vi "Main.vi"(0 "Search Bar":string(combo), 1 "Copy":bool, 2 "Expand/Collapse All":bool, 5 "Tree":string[](tree), 7 "Top Level folder path":path, 11 "Error In":errorcluster) -> (4 "Path":path, 6 "Report String":string, 15 "Error Out":errorcluster)   [LabVIEW 2019]
doc: "Implements a file explorer interface to display folders and files, displaying attributes and supporting operations like selection, copying, sorting and report generation about the folders."
uses:
  Controls/Queue Operation.ctl
  Controls/Queue Element.ctl
  Controls/File explorer Data.ctl
  Controls/Item.ctl
  <vilib>/Utility/miscctls.llb/LVPoint32TypeDef.ctl
  49cb5066-c8fb-45b1-b1e9-3b55b32f25bf.vi
  Controls/Error Details.ctl
panel:
  # "Instructions:\n1. Run the VI.\n2. Specify the top-level folder path and view the folder structure along with its attributes in the tree control.\n3. Tree headers acts as sorting triggers.\n4. Click the checkbox next to folder to select or deselect it. View the generated report for the checked folders in the report string.\n5. Press the Expand/Collapse button to expand/collapse all the items in the tree.\n6. Enter the folder name in the search bar to expand all the nodes that match the searched keyword.\n7. Select the files and click on the copy to copy the files in the desired destination.\n8. Click Panel Close to stop the VI."
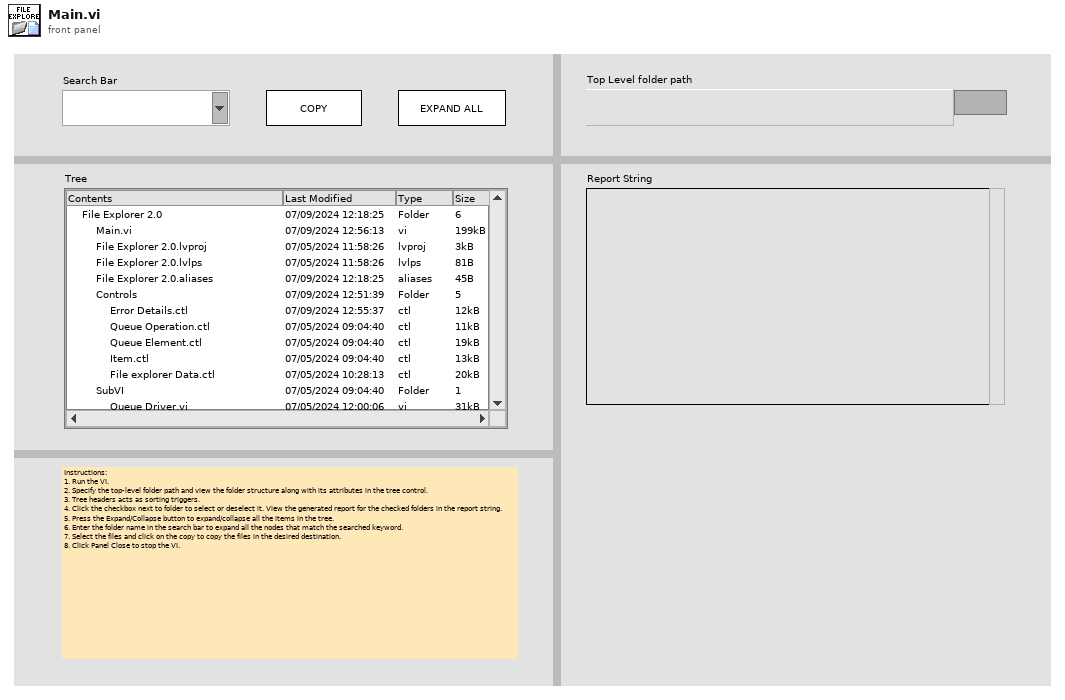
[diagram p1: front panel]
types:
  T1 = typedef "Queue Element.ctl" = cluster{"State":string, "Data":variant}
  T2 = typedef "File explorer Data.ctl" = cluster{"Path In":path, "Indent":i32, "All Folders":path[], "All Files":path[], "Folder Items":T3[], "File Items":T3[], "Selected tags":string[], "Report String":string, "Search String":string, "Search Results":string[], "Checked Folders":string[], "Files Selected":string[], "Stop Event":refnum<user-event>, "Sort Header":i32, "Time Flag":i16, "Type Flag":i16, "Size Flag":i16, "Reverse?":bool, "New Folder Path":path, "Expand?":bool, "Open? State":bool[], "Nodes":path[], "Active Tag":string, "Repopulate?":bool}
  T3 = typedef "Item.ctl" = cluster{"Left Cell String":string, "Child Text":string[], "Child Tag":string, "Child Only?":bool, "Parent Tag":string, "Item Indent":i32}
  T4 = typedef "Queue Operation.ctl" = enum16{"Create and Enqueue N", "Enqueue", "Enqueue N", "Dequeue", "Enstack N", "Flush", "Release"}
  T5 = typedef "LVPoint32TypeDef.ctl" = cluster{"Horizontal":i32, "Vertical":i32}
  T6 = typedef "Error Details.ctl" = errorcluster
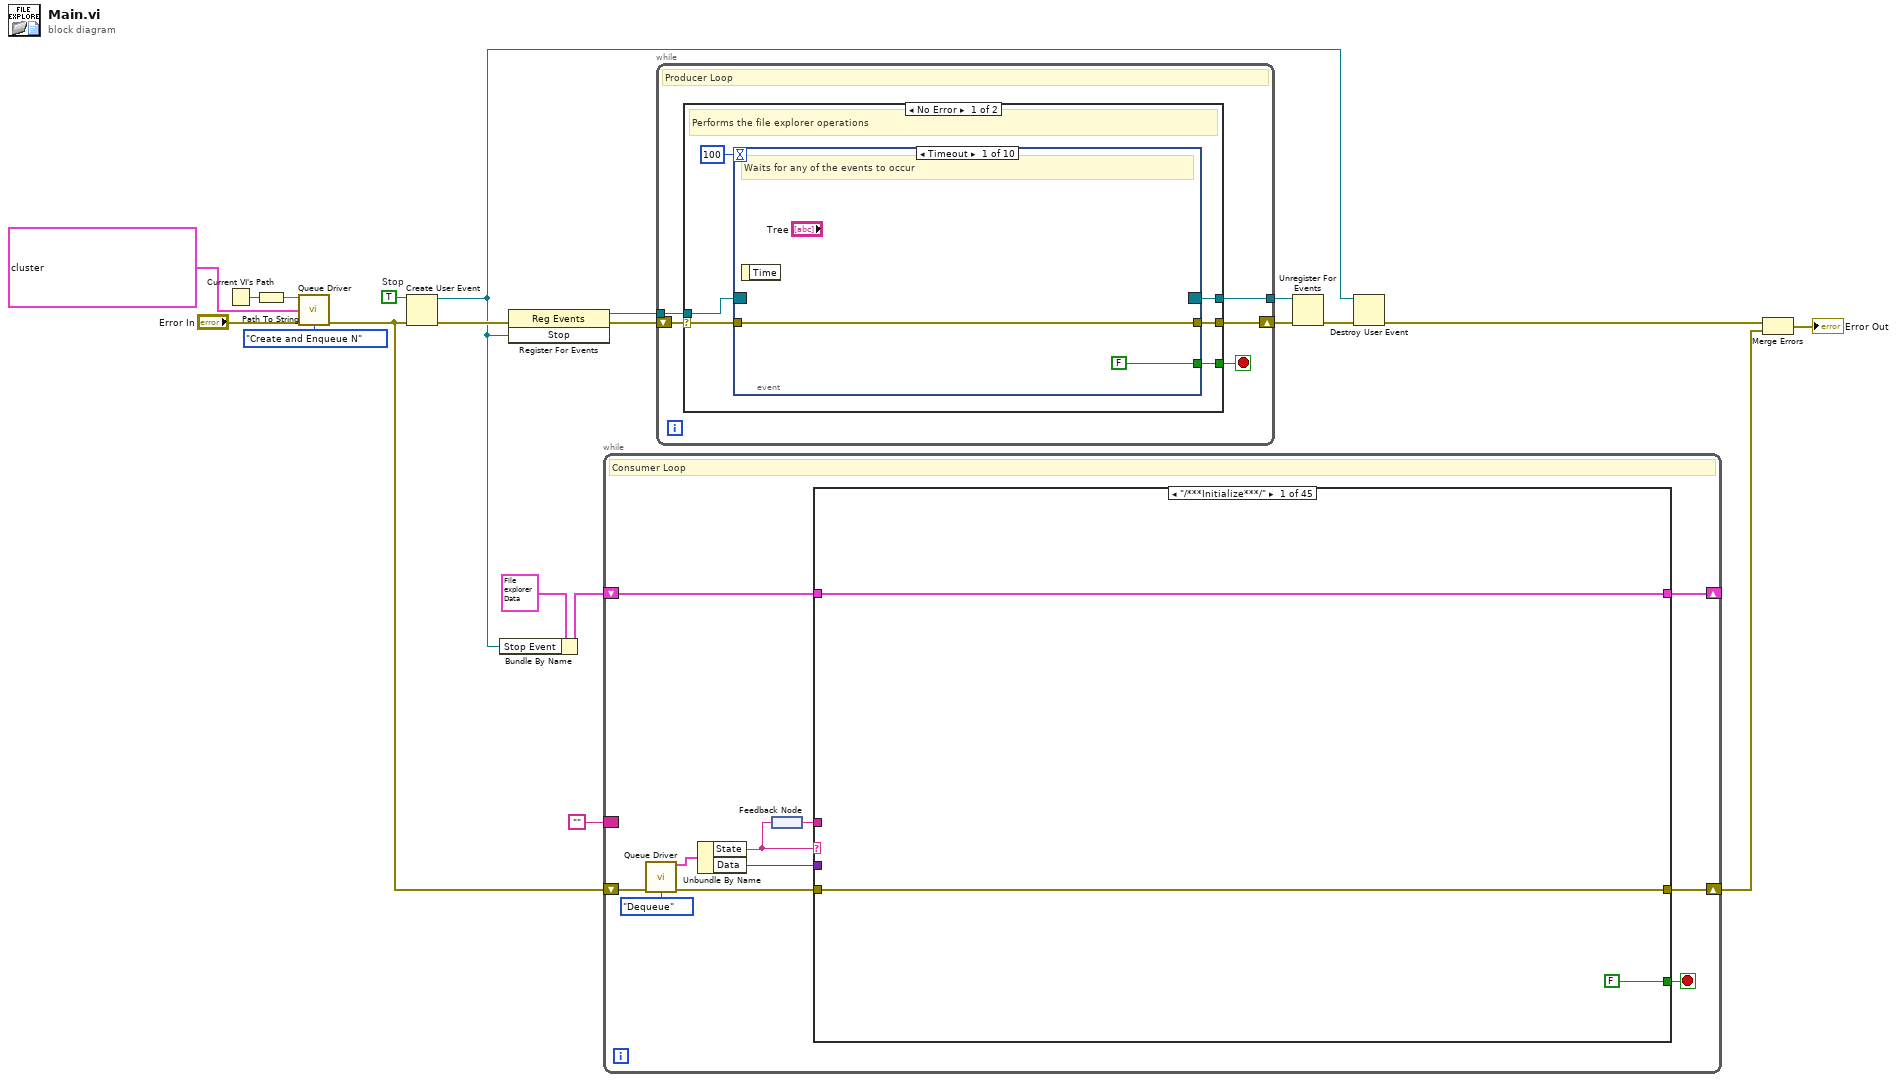
[diagram p0: block diagram]
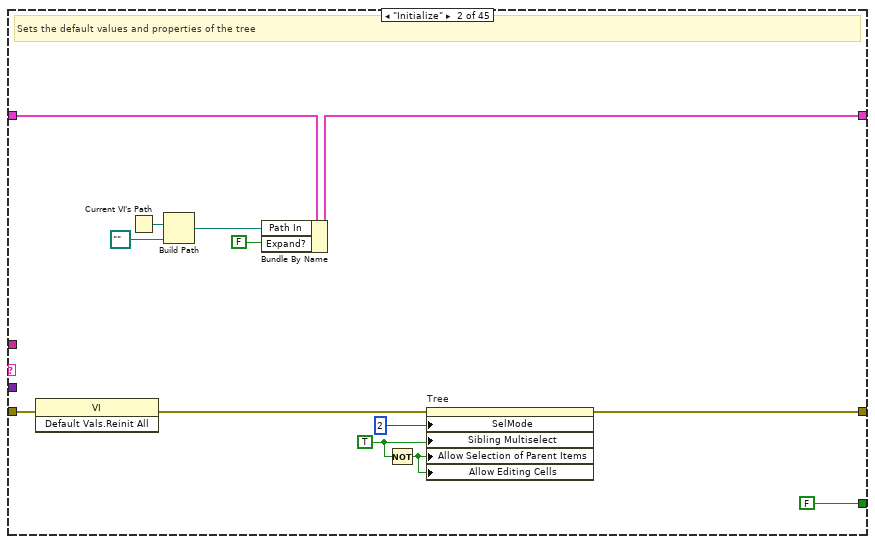
[diagram p2: hidden frame]
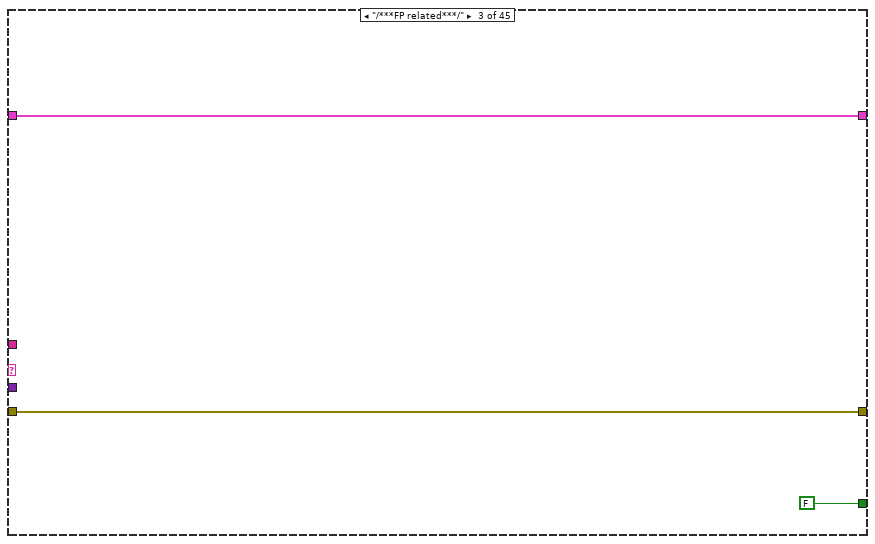
[diagram p3: hidden frame]
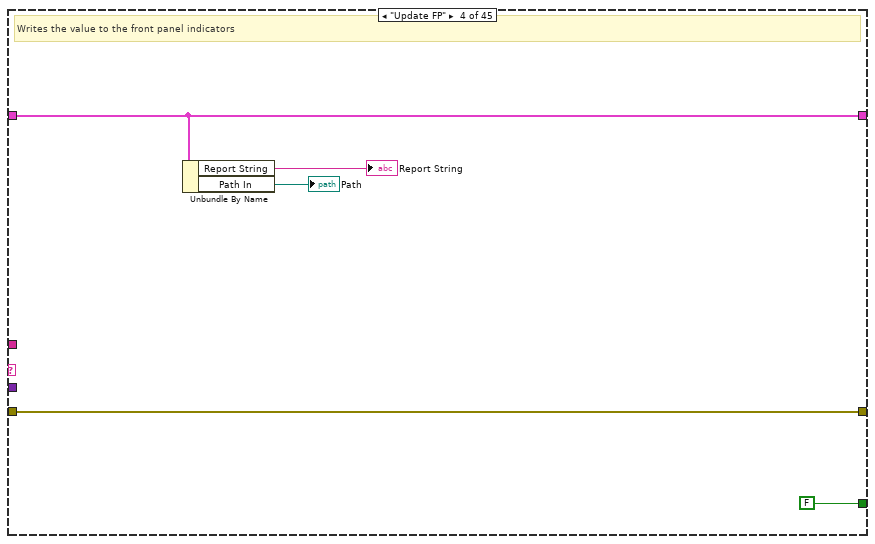
[diagram p4: hidden frame]
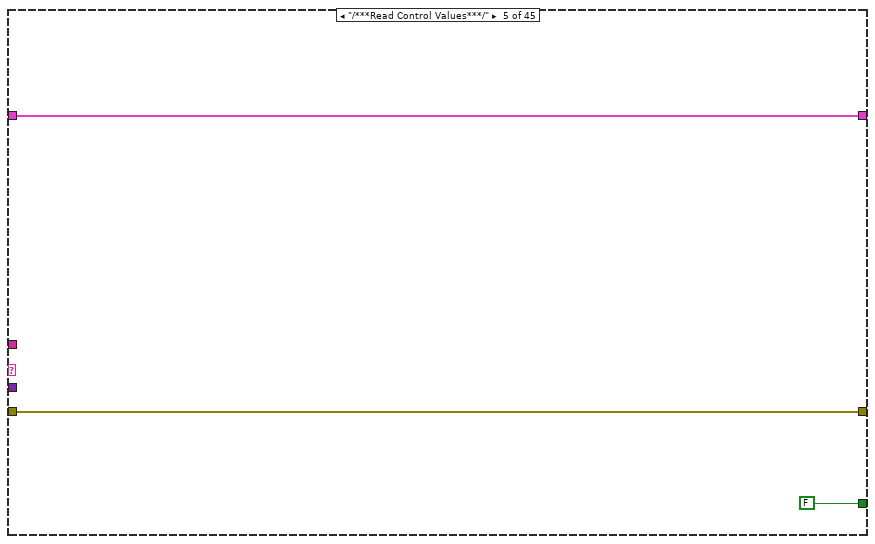
[diagram p5: hidden frame]
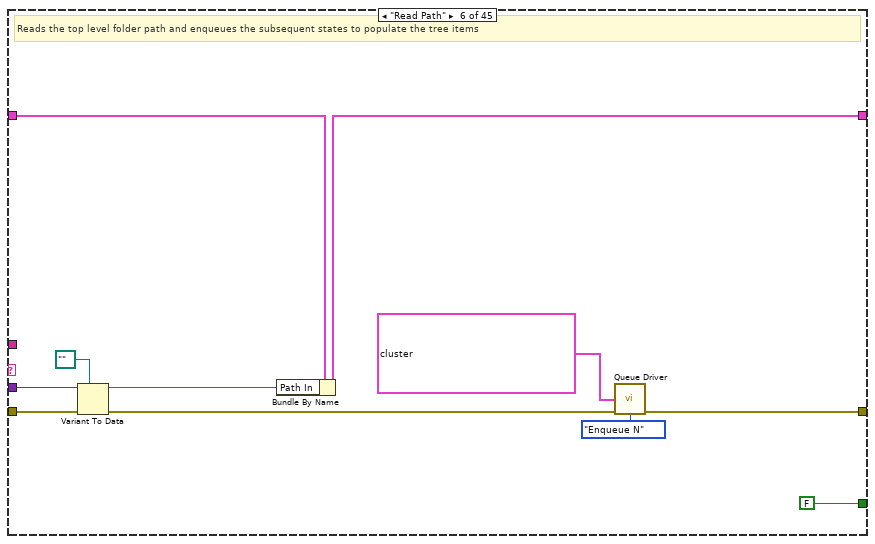
[diagram p6: hidden frame]
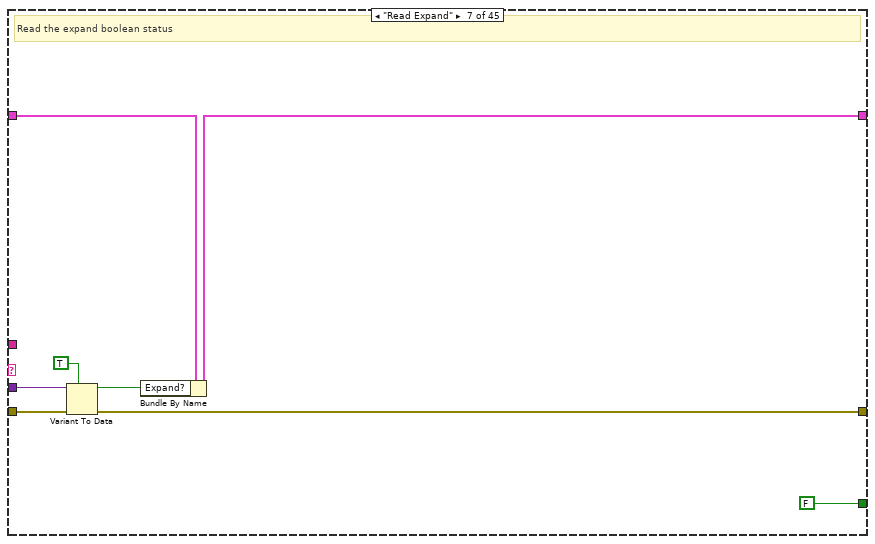
[diagram p7: hidden frame]
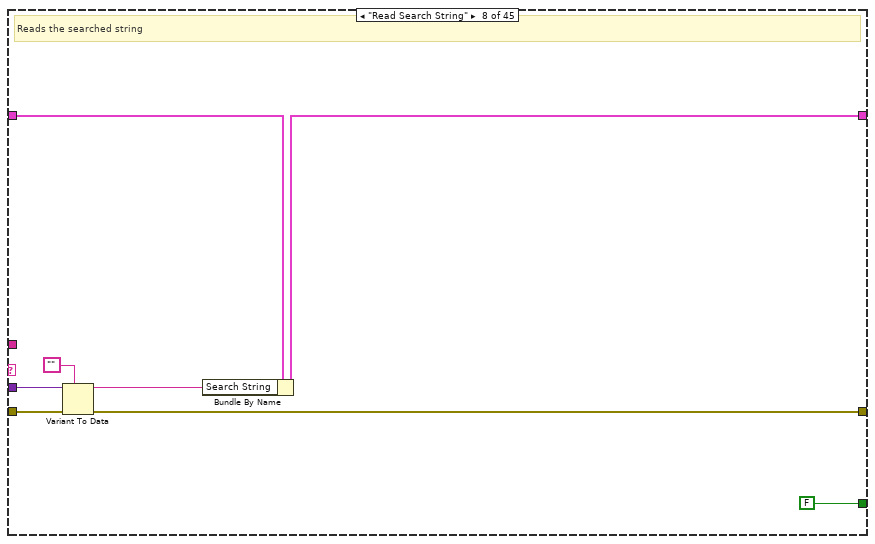
[diagram p8: hidden frame]
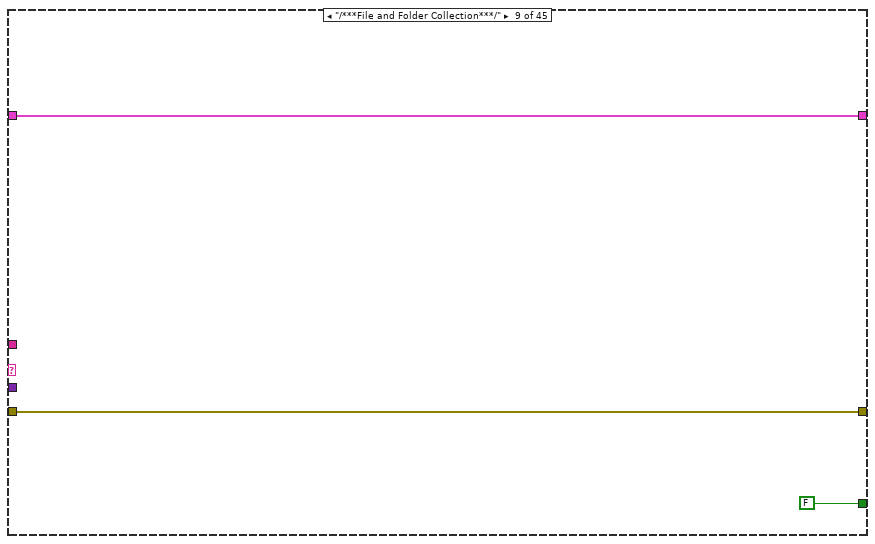
[diagram p9: hidden frame]
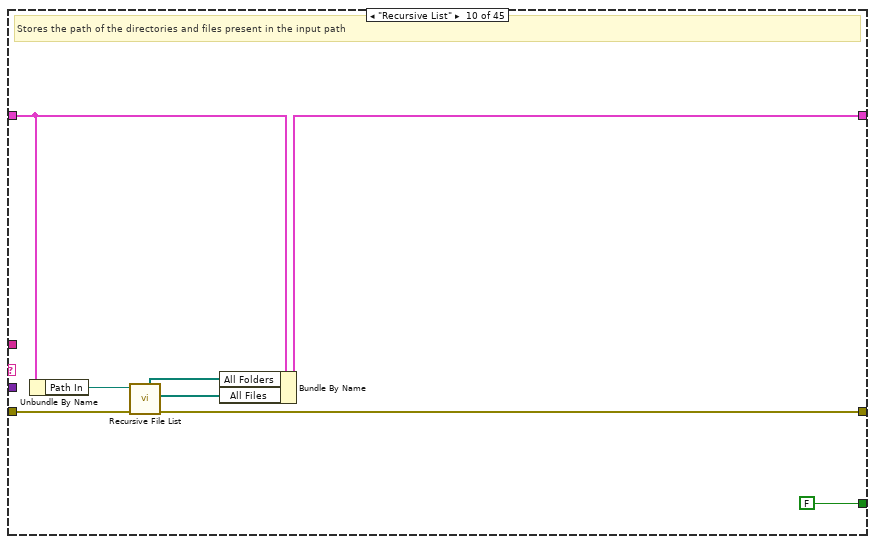
[diagram p10: hidden frame]
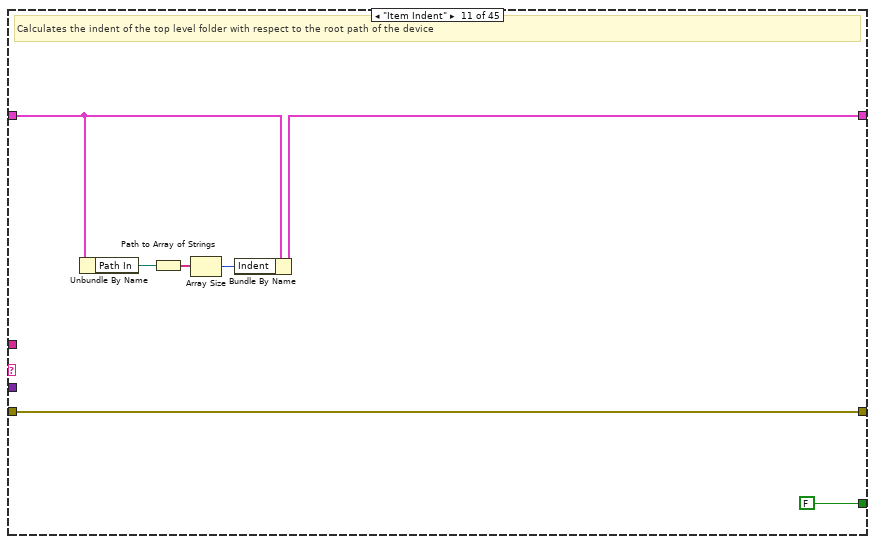
[diagram p11: hidden frame]
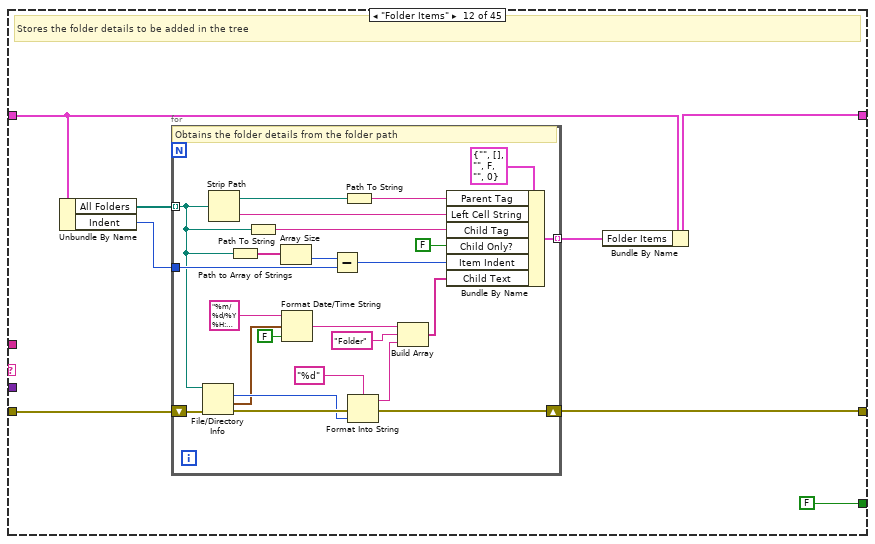
[diagram p12: hidden frame]
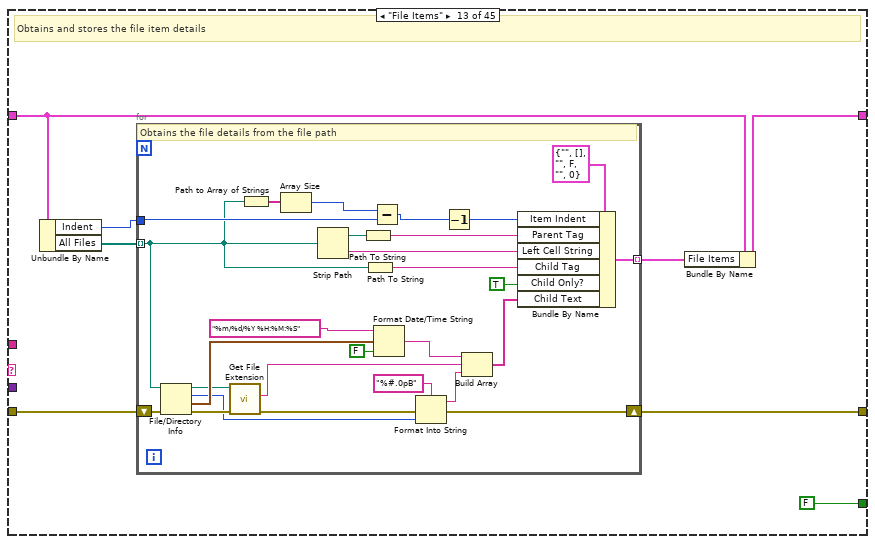
[diagram p13: hidden frame]
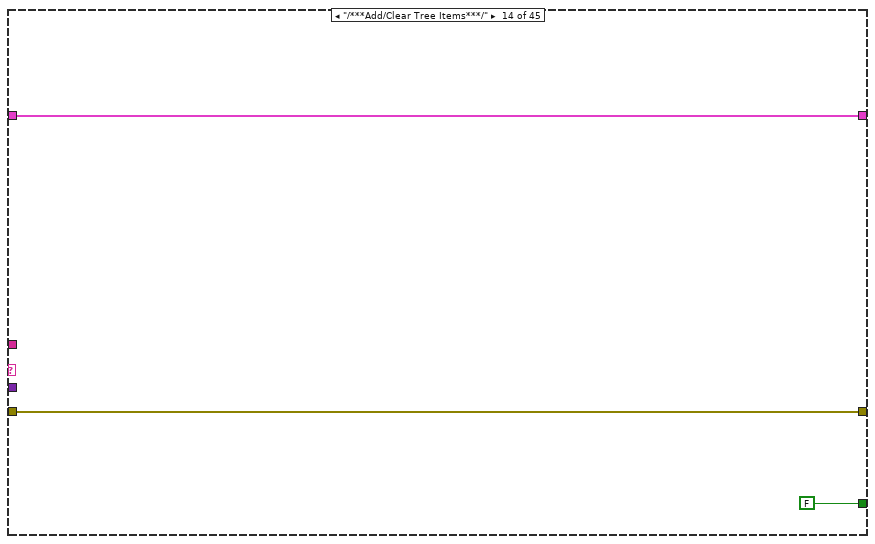
[diagram p14: hidden frame]
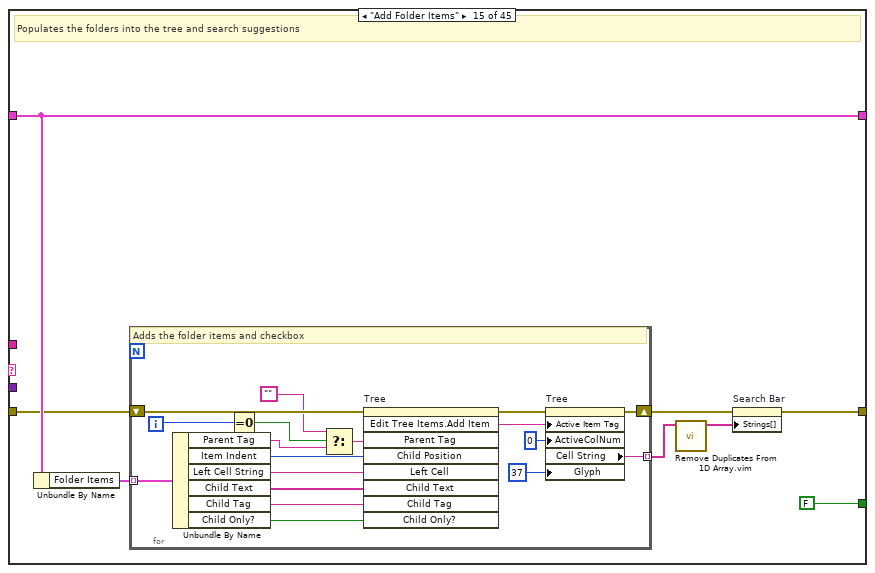
[diagram p15: hidden frame]
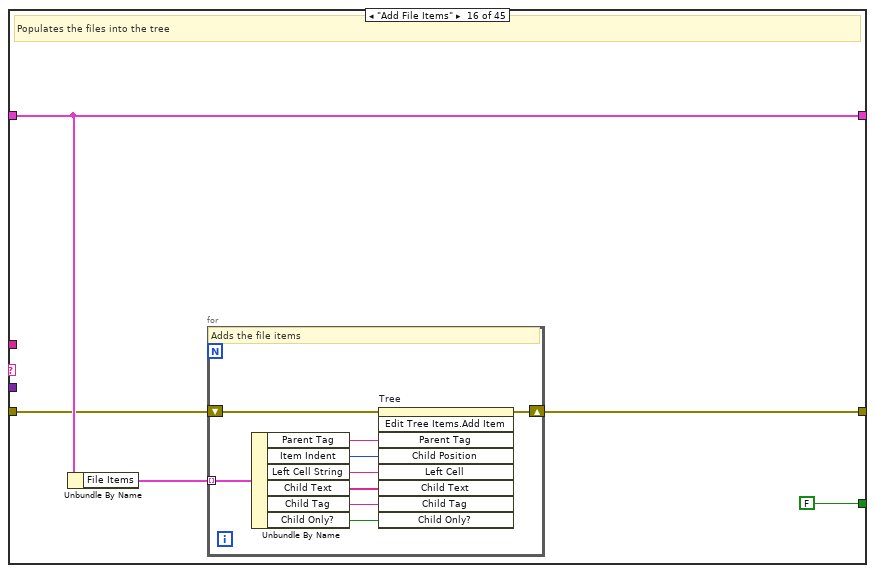
[diagram p16: hidden frame]
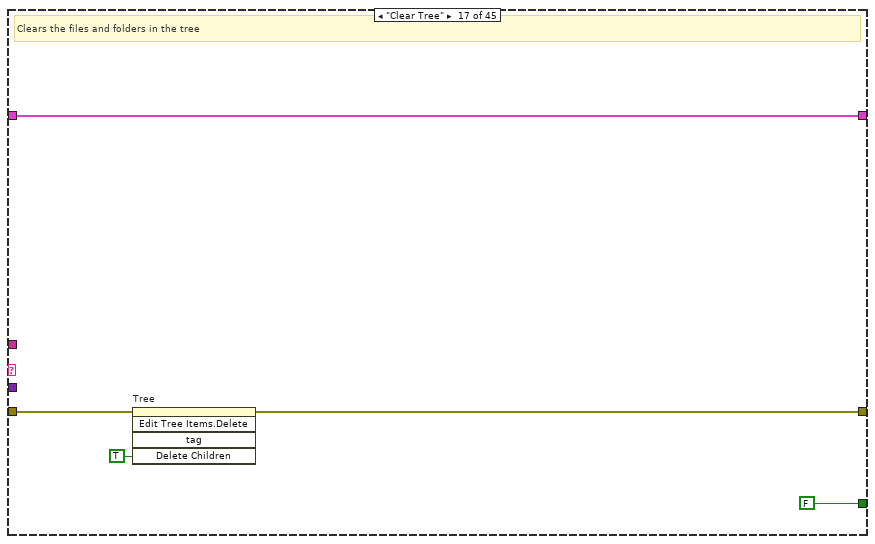
[diagram p17: hidden frame]
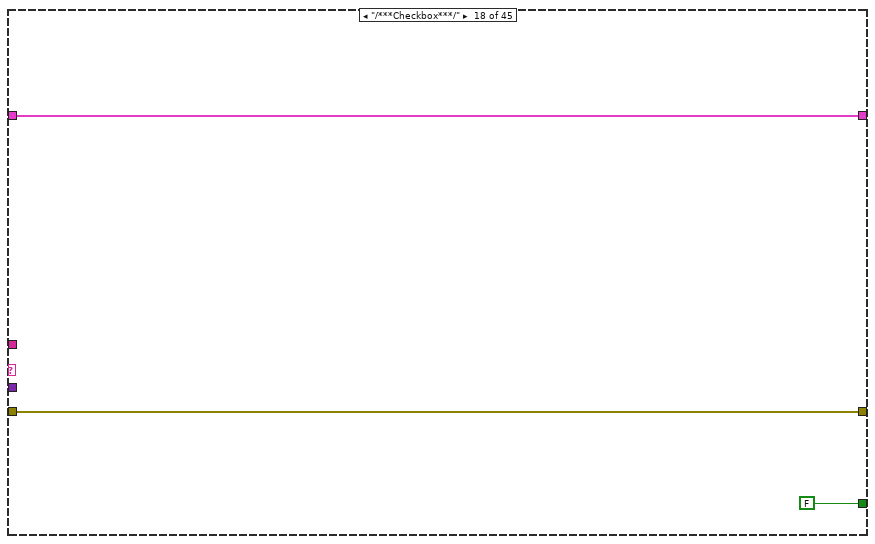
[diagram p18: hidden frame]
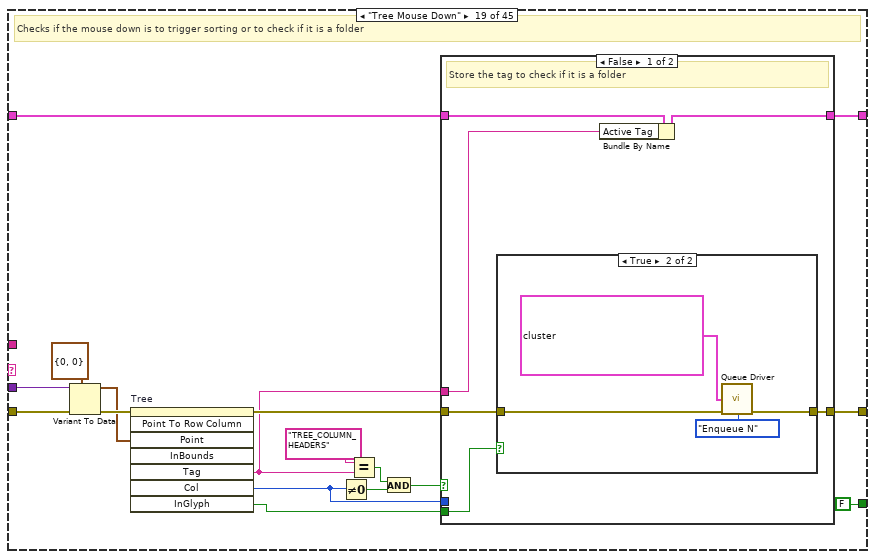
[diagram p19: hidden frame]
diagram:
  w11 = TRUE  # Stop
  n1 = Current VI's Path() -> (path=w3:path)
  n2 = Path To String(path=w3) -> (string=w2:string)
  n3 = call "Queue Driver.vi"("Queue Name"=w2, "Array of Elements"=T1[] [{"State"="Initialize", "Data"=variant}, {"State"="Update FP", "Data"=variant}, {"State"="Clear Tree", "Data"=variant}, {"State"="Recursive List", "Data"=variant}, {"State"="Item Indent", "Data"=variant}, {"State"="Folder Items", "Data"=variant}, {"State"="File Items", "Data"=variant}, {"State"="Add Folder Items", "Data"=variant}, {"State"="Expand or Collapse", "Data"=variant}, {"State"="Add File Items", "Data"=variant}], "Error In"="Error In", "Queue Operation"=Queue_Operation."Create and Enqueue N") -> ("Error Out"=w17:errorcluster)  [unwired: 10 in, 1 out]
  n4 = Create User Event(user event datatype=w11, error in=w17) -> (user event=w4:refnum<user-event>, error out=w12:errorcluster)
  n5 = Bundle By Name(cluster=T2 {"Path In"=path "", "Indent"=0, "All Folders"=[], "All Files"=[], "Folder Items"=[], "File Items"=[], "Selected tags"=[], "Report String"="", "Search String"="", "Search Results"=[], "Checked Folders"=[], "Files Selected"=[], "Stop Event"=refnum, "Sort Header"=0, "Time Flag"=0, "Type Flag"=0, "Size Flag"=0, "Reverse?"=TRUE, "New Folder Path"=path "", "Expand?"=TRUE, "Open? State"=[], "Nodes"=[], "Active Tag"="", "Repopulate?"=TRUE}, "Stop Event"=w4) -> (w5:T2)
  n6 = register-events(error in=w12, w4) -> (reference out=w10:refnum<event-registration>, error out=w20:errorcluster)  [unwired: 1 in]
  n7 = while {
    border: "" ("State") -> [_]
    shift-right: [w31] -> w13
    shift-left: w17 -> [w30]
    shift-right: [w23] -> _
    shift-left: w5 -> [w24]
    stop <- w22 stop-if-true
    # "Consumer Loop"
    n8 = call "Queue Driver.vi"("Error In"=w30, "Queue Operation"=Queue_Operation."Dequeue") -> ("Dequeue Element"=w21:T1, "Error Out"=w29:errorcluster)  [unwired: 12 in]
    n9 = Unbundle By Name(w21) -> ("State"=w27:string, "Data"=w28:variant)
    n10 = feedback-in #1(w27) -> ()
    n11 = feedback #1() -> (w26:string)
    n12 = case shown="\"/***Initialize***/\"" w27 {
      tunnel: w29 -> [w34 w47 w50 w55 w58 w69 w76 w85 w88 w94 w103 w108 w142 w173 w179 w203 w218 w221 w238 w265 w279 w285 w298 w318 w325 w345 w355 w363 w367 w383 w396 w447 w457 w469 w503 w506 w514 w522 w534 w537 w544 w568 w580 w590 w594]
      tunnel: [w34 w35 w50 w55 w58 w65 w75 w83 w88 w91 w103 w107 w141 w173 w176 w202 w216 w221 w224 w264 w279 w286 w297 w318 w320 w341 w355 w357 w366 w381 w395 w440 w457 w459 w502 w506 w513 w525 w533 w537 w540 w565 w580 w584 w594] -> w31
      tunnel: w28 -> [_ _ _ _ _ w68 w74 w82 _ _ _ _ _ _ _ _ _ _ w237 _ _ _ _ _ _ _ _ w362 _ _ _ _ _ w467 _ _ _ _ _ _ _ w559 _ _ _]
      tunnel: w26 -> [_ _ _ _ _ _ _ _ _ _ _ _ _ _ _ _ _ _ _ _ _ _ _ _ _ _ _ _ _ _ _ _ _ _ _ _ _ _ _ _ w543 _ _ _ _]
      tunnel: w24 -> [w33 w46 w49 w54 w57 w63 w77 w84 w87 w96 w102 w105 w143 w172 w181 w204 w217 w220 w223 w262 w278 w284 w302 w317 w328 w347 w354 w359 w369 w382 w391 w449 w456 w464 w499 w505 w512 w524 w532 w536 w539 w564 w579 w583 w592]
      tunnel: [w33 w44 w49 w54 w57 w62 w72 w80 w87 w93 w99 w104 w140 w172 w181 w204 w217 w220 w222 w262 w278 w282 w300 w317 w326 w347 w354 w360 w369 w379 w390 w449 w456 w465 w499 w505 w510 w524 w532 w536 w539 w564 w579 w583 w592] -> w23
      tunnel: [FALSE FALSE FALSE FALSE FALSE FALSE FALSE FALSE FALSE FALSE FALSE FALSE FALSE FALSE FALSE FALSE FALSE FALSE FALSE FALSE FALSE FALSE FALSE FALSE FALSE FALSE FALSE FALSE FALSE FALSE FALSE FALSE FALSE FALSE FALSE FALSE FALSE FALSE FALSE FALSE FALSE FALSE FALSE TRUE FALSE] -> w22
      frame "/***Initialize***/" {
      }
      frame "Initialize" {
        w37 = TRUE ("Sibling Multiselect")
        # "Sets the default values and properties of the tree"
        n13 = invoke on="Invoke Node" class="VI" method="Default Vals.Reinit All"(error in=w47) -> (error out=w41:errorcluster)  [unwired: 2 in, 2 out]
        n14 = Current VI's Path() -> (path=w43:path)
        n15 = Build Path(base path=w43, name or relative path=path "..") -> (appended path=w40:path)
        n16 = Bundle By Name(cluster=w46, "Path In"=w40, "Expand?"=FALSE) -> (w44:T2)
        n17 = Not(x=w37) -> (.not. x?=w36:bool)
        n18 = property on="Tree" class="Tree (strict)"(error in=w41, "SelMode"=2 ("Selection Mode"), "Sibling Multiselect"=w37, "Allow Selection of Parent Items"=w36, "Allow Editing Cells"=w36) -> (error out=w35:errorcluster)  [unwired: 1 in, 1 out]
      }
      frame "/***FP related***/" {
      }
      frame "Update FP" {
        # "Writes the value to the front panel indicators"
        n19 = Unbundle By Name(w54) -> ("Report String"=→"Report String":string, "Path In"=→"Path":path)
      }
      frame "/***Read Control Values***/" {
      }
      frame "Read Path" {
        # "Reads the top level folder path and enqueues the subsequent states to populate the tree items"
        n20 = Variant To Data(error in=w69, type=path "", Variant=w68) -> (data=w61:path, error out=w66:errorcluster)
        n21 = Bundle By Name(cluster=w63, "Path In"=w61) -> (w62:T2)
        n22 = call "Queue Driver.vi"("Array of Elements"=T1[] [{"State"="Update FP", "Data"=variant}, {"State"="Clear Tree", "Data"=variant}, {"State"="Recursive List", "Data"=variant}, {"State"="Item Indent", "Data"=variant}, {"State"="Folder Items", "Data"=variant}, {"State"="File Items", "Data"=variant}, {"State"="Add Folder Items", "Data"=variant}, {"State"="Expand or Collapse", "Data"=variant}, {"State"="Add File Items", "Data"=variant}], "Error In"=w66, "Queue Operation"=Queue_Operation."Enqueue N") -> ("Error Out"=w65:errorcluster)  [unwired: 11 in, 1 out]
      }
      frame "Read Expand" {
        # "Read the expand boolean status"
        n23 = Variant To Data(error in=w76, type=TRUE, Variant=w74) -> (data=w71:bool, error out=w75:errorcluster)
        n24 = Bundle By Name(cluster=w77, "Expand?"=w71) -> (w72:T2)
      }
      frame "Read Search String" {
        # "Reads the searched string"
        n25 = Variant To Data(error in=w85, type="" ("Search Bar"), Variant=w82) -> (data=w79:string, error out=w83:errorcluster)
        n26 = Bundle By Name(cluster=w84, "Search String"=w79) -> (w80:T2)
      }
      frame "/***File and Folder Collection***/" {
      }
      frame "Recursive List" {
        # "Stores the path of the directories and files present in the input path"
        n27 = Unbundle By Name(w96) -> ("Path In"=w95:path)
        n28 = call <vilib>:"Recursive File List.vi"("error in (no error)"=w94, "Folder Path"=w95) -> ("error out"=w91:errorcluster, "All Files in Dir"=w92:path[], "All Folders"=w89:path[])  [unwired: 5 in, 2 out]
        n29 = Bundle By Name(cluster=w96, "All Folders"=w89, "All Files"=w92) -> (w93:T2)
      }
      frame "Item Indent" {
        # "Calculates the indent of the top level folder with respect to the root path of the device"
        n30 = Unbundle By Name(w102) -> ("Path In"=w101:path)
        n31 = Path to Array of Strings(0:w101) -> (2:w100:string[])  [unwired: 1 out]
        n32 = Array Size(array=w100) -> (size(s)=w98:i32)
        n33 = Bundle By Name(cluster=w102, "Indent"=w98) -> (w99:T2)
      }
      frame "Folder Items" {
        # "Stores the folder details to be added in the tree"
        n34 = Unbundle By Name(w105) -> ("All Folders"=w111:path[], "Indent"=w110:i32)
        n35 = for {
          tunnel: [w135] -> w109 mode=indexing
          tunnel: w111 -> [w115] mode=indexing
          tunnel: w110 -> [w131]
          shift-right: [w122] -> w107
          shift-left: w108 -> [w123]
          # "Obtains the folder details from the folder path"
          n36 = File/Directory Info(path=w115, error in=w123) -> (size=w129:i64, last mod=w126:timestamp, error out=w130:errorcluster)  [unwired: 4 out]
          n37 = Strip Path(path=w115) -> (stripped path=w113:path, name=w132:string)
          n38 = Path to Array of Strings(0:w115) -> (2:w134:string[])  [unwired: 1 out]
          n39 = Path To String(path=w115) -> (string=w119:string)
          n40 = Array Size(array=w134) -> (size(s)=w133:i32)
          n41 = Format Date/Time String(time format string (%c)="%m/%d/%Y %H:%M:%S", seconds (now)=w126, UTC format=FALSE) -> (date/time string=w124:string)
          n42 = Subtract(x=w133, y=w131) -> (x-y=w118:i32)
          n43 = Path To String(path=w113) -> (string=w112:string)
          n44 = Format Into String(format string="%d", error in=w130, w129) -> (resulting string=w120:string, error out=w122:errorcluster)  [unwired: 1 in]
          n45 = Build Array(w124, "Folder" ("element"), w120) -> (w121:string[])
          n46 = Bundle By Name(cluster=T3 {"Left Cell String"="", "Child Text"=[], "Child Tag"="", "Child Only?"=FALSE, "Parent Tag"="", "Item Indent"=0} ("Item"), "Parent Tag"=w112, "Left Cell String"=w132, "Child Tag"=w119, "Child Only?"=FALSE, "Item Indent"=w118, "Child Text"=w121) -> (w135:T3)
        }
        n47 = Bundle By Name(cluster=w105, "Folder Items"=w109) -> (w104:T2)
      }
      frame "File Items" {
        # "Obtains and stores the file item details"
        n48 = Unbundle By Name(w143) -> ("Indent"=w137:i32, "All Files"=w139:path[])
        n49 = for {
          tunnel: [w161] -> w138 mode=indexing
          shift-right: [w155] -> w141
          shift-left: w142 -> [w170]
          tunnel: w139 -> [w148] mode=indexing
          tunnel: w137 -> [w153]
          # "Obtains the file details from the file path"
          n50 = File/Directory Info(path=w148, error in=w170) -> (path out=w149:path, size=w152:i64, last mod=w166:timestamp, error out=w169:errorcluster)  [unwired: 3 out]
          n51 = call <vilib>:"Get File Extension.vi"("error in (no error)"=w169, "file"=w149) -> ("error out"=w145:errorcluster, "lowercase file extension"=w144:string)  [unwired: 5 in, 3 out]
          n52 = Path to Array of Strings(0:w148) -> (2:w160:string[])  [unwired: 1 out]
          n53 = Array Size(array=w160) -> (size(s)=w154:i32)
          n54 = Strip Path(path=w148) -> (stripped path=w159:path, name=w162:string)
          n55 = Path To String(path=w159) -> (string=w157:string)
          n56 = Path To String(path=w148) -> (string=w156:string)
          n57 = Subtract(x=w154, y=w153) -> (x-y=w146:i32)
          n58 = Format Date/Time String(time format string (%c)="%m/%d/%Y %H:%M:%S", seconds (now)=w166, UTC format=FALSE) -> (date/time string=w158:string)
          n59 = Format Into String(format string="%#.0pB", error in=w145, w152) -> (resulting string=w151:string, error out=w155:errorcluster)  [unwired: 1 in]
          n60 = Decrement(x=w146) -> (x-1=w147:i32)
          n61 = Build Array(w158, w144, w151) -> (w150:string[])
          n62 = Bundle By Name(cluster=T3 {"Left Cell String"="", "Child Text"=[], "Child Tag"="", "Child Only?"=FALSE, "Parent Tag"="", "Item Indent"=0} ("Item"), "Item Indent"=w147, "Parent Tag"=w157, "Left Cell String"=w162, "Child Tag"=w156, "Child Only?"=TRUE, "Child Text"=w150) -> (w161:T3)
        }
        n63 = Bundle By Name(cluster=w143, "File Items"=w138) -> (w140:T2)
      }
      frame "/***Add/Clear Tree Items***/" {
      }
      frame "Add Folder Items" {
        # "Populates the folders into the tree and search suggestions"
        n64 = Unbundle By Name(w181) -> ("Folder Items"=w178:T3[])
        n65 = for {
          shift-right: [w192] -> w177
          shift-left: w179 -> [w199]
          tunnel: w178 -> [w198] mode=indexing
          tunnel: [w190] -> w175 mode=indexing
          i -> [w182]
          # "Adds the folder items and checkbox"
          n66 = Unbundle By Name(w198) -> ("Parent Tag"=w186:string, "Item Indent"=w187:i32, "Left Cell String"=w196:string, "Child Text"=w195:string[], "Child Tag"=w194:string, "Child Only?"=w197:bool)
          n67 = Equal To 0?(x=w182) -> (x = 0?=w183:bool)
          n68 = Select(t="", s=w183, f=w186) -> (s? t:f=w185:string)
          n69 = invoke on="Tree" class="Tree (strict)" method="Edit Tree Items.Add Item"(error in=w199, "Parent Tag"=w185, "Child Position"=w187, "Left Cell"=w196, "Child Text"=w195, "Child Tag"=w194, "Child Only?"=w197) -> (error out=w193:errorcluster, "Edit Tree Items:Add Item"=w191:string)  [unwired: 2 in, 7 out]
          n70 = property on="Tree" class="Tree (strict)"(error in=w193, "Active Item Tag"=w191, "ActiveColNum"=0 ("Active Cell:Active Column Number"), "Glyph"=37 ("Active Item:Symbol Index")) -> (error out=w192:errorcluster, "Cell String"=w190:string)  [unwired: 1 in, 1 out]
        }
        n71 = call "Remove Duplicates From 1D Array.vim"("array"=w175) -> ("array with duplicates removed"=w174:string[])  [unwired: 10 in]
        n72 = property on="Search Bar" class="CmbBox"(error in=w177, "Strings[]"=w174) -> (error out=w176:errorcluster)  [unwired: 1 in, 1 out]
      }
      frame "Add File Items" {
        # "Populates the files into the tree"
        n73 = Unbundle By Name(w204) -> ("File Items"=w201:T3[])
        n74 = for {
          shift-right: [w212] -> w202
          shift-left: w203 -> [w213]
          tunnel: w201 -> [w211] mode=indexing
          # "Adds the file items"
          n75 = Unbundle By Name(w211) -> ("Parent Tag"=w206:string, "Item Indent"=w205:i32, "Left Cell String"=w209:string, "Child Text"=w208:string[], "Child Tag"=w207:string, "Child Only?"=w210:bool)
          n76 = invoke on="Tree" class="Tree (strict)" method="Edit Tree Items.Add Item"(error in=w213, "Parent Tag"=w206, "Child Position"=w205, "Left Cell"=w209, "Child Text"=w208, "Child Tag"=w207, "Child Only?"=w210) -> (error out=w212:errorcluster)  [unwired: 2 in, 8 out]
        }
      }
      frame "Clear Tree" {
        # "Clears the files and folders in the tree"
        n77 = invoke on="Tree" class="Tree (strict)" method="Edit Tree Items.Delete"(error in=w218, "Delete Children"=TRUE ("Sibling Multiselect")) -> (error out=w216:errorcluster)  [unwired: 3 in, 4 out]
      }
      frame "/***Checkbox***/" {
      }
      frame "Tree Mouse Down" {
        # "Checks if the mouse down is to trigger sorting or to check if it is a folder"
        n78 = Variant To Data(error in=w238, type=T5 {"Horizontal"=0, "Vertical"=0} ("Coords"), Variant=w237) -> (data=w234:T5, error out=w235:errorcluster)
        n79 = invoke on="Tree" class="Tree (strict)" method="Point To Row Column"(error in=w235, "Point"=w234) -> (error out=w230:errorcluster, "Tag"=w225:string, "Col"=w228:i32, "InGlyph"=w226:bool)  [unwired: 6 in, 4 out]
        n80 = Not Equal To 0?(x=w228) -> (x != 0?=w231:bool)
        n81 = Equal?(x="TREE_COLUMN_HEADERS", y=w225) -> (x = y?=w232:bool)
        n82 = And(x=w232, y=w231) -> (x .and. y?=w229:bool)
        n83 = case shown="False" w229 {
          tunnel: w230 -> [w243 w253]
          tunnel: [w242 w252] -> w224
          tunnel: w228 -> [_ w256]
          tunnel: w226 -> [w241 _]
          tunnel: w225 -> [w239 _]
          tunnel: w223 -> [w244 w250]
          tunnel: [w240 w250] -> w222
          frame False {
            # "Store the tag to check if it is a folder"
            n84 = case shown="True" w241 {
              tunnel: w243 -> [w245 w248]
              tunnel: [w245 w247] -> w242
              frame False {
              }
              frame True {
                n85 = call "Queue Driver.vi"("Array of Elements"=T1[] [{"State"="Toggle Checkbox", "Data"=variant}, {"State"="Selected Folders", "Data"=variant}, {"State"="Folder Details", "Data"=variant}, {"State"="Update FP", "Data"=variant}], "Error In"=w248, "Queue Operation"=Queue_Operation."Enqueue N") -> ("Error Out"=w247:errorcluster)  [unwired: 11 in, 1 out]
              }
            }
            n86 = Bundle By Name(cluster=w244, "Active Tag"=w239) -> (w240:T2)
          }
          frame True {
            # "Triggers the Sort"
            n87 = To Variant(anything=w256) -> (Variant=w259:variant)
            n88 = Bundle By Name(cluster=T1 {"State"="", "Data"=variant} ("Enqueue Element"), "Data"=w259, "State"="Sort Type") -> (w260:T1)
            n89 = Build Array(w260, T1 {"State"="Sort", "Data"=variant} ("element")) -> (w251:T1[])
            n90 = call "Queue Driver.vi"("Array of Elements"=w251, "Error In"=w253, "Queue Operation"=Queue_Operation."Enqueue N") -> ("Error Out"=w252:errorcluster)  [unwired: 11 in, 1 out]
          }
        }
      }
      frame "Toggle Checkbox" {
        # "Toggles the checkbox if selected item is a folder"
        n91 = Unbundle By Name(w262) -> ("Active Tag"=w261:string)
        n92 = property on="Tree" class="Tree (strict)"(error in=w265, "Active Item Tag"=w261) -> (error out=w268:errorcluster, "Glyph"=w267:i32, "Child-Only?"=w266:bool)  [unwired: 1 in, 1 out]
        n93 = case shown="False" w266 {
          tunnel: [w275 w276] -> w264
          tunnel: w268 -> [w274 w276]
          tunnel: w267 -> [w269 _]
          frame False {
            w271 = 37 ("x")
            # "Toggles the checkbox"
            n94 = Equal?(x=w269, y=w271) -> (x = y?=w272:bool)
            n95 = Increment(x=w269) -> (x+1=w270:i32)
            n96 = Select(t=w270, s=w272, f=w271) -> (s? t:f=w273:i32)
            n97 = property on="Tree" class="Tree (strict)"(error in=w274, "Glyph"=w273) -> (error out=w275:errorcluster)  [unwired: 1 in, 1 out]
          }
          frame True {
          }
        }
      }
      frame "/***Report Generation***/" {
      }
      frame "Selected Folders" {
        # "Stores the folders in which checkbox is ticked"
        n98 = Unbundle By Name(w284) -> ("All Folders"=w283:path[])
        n99 = for {
          shift-right: [w293] -> w286
          shift-left: w285 -> [w294]
          tunnel: w283 -> [w292] mode=indexing
          tunnel: [w289] -> w280 mode=indexing if=w290
          # "separates the checked folders based on the symbol index"
          n100 = Path To String(path=w292) -> (string=w291:string)
          n101 = property on="Tree" class="Tree (strict)"(error in=w294, "Active Item Tag"=w291) -> (error out=w293:errorcluster, "Active Item Tag"=w289:string, "Glyph"=w288:i32)  [unwired: 1 in, 1 out]
          n102 = Equal?(x=w288, y=38 ("x")) -> (x = y?=w290:bool)
        }
        n103 = Bundle By Name(cluster=w284, "Checked Folders"=w280) -> (w282:T2)
      }
      frame "Folder Details" {
        # "Obtains the details of the checked folders and prepares the report string"
        n104 = Unbundle By Name(w302) -> ("Checked Folders"=w301:string[])
        n105 = for {
          tunnel: w301 -> [w309] mode=indexing
          shift-right: [w313] -> w297
          shift-left: w298 -> [w315]
          tunnel: [w307] -> w296 mode=indexing
          w305 = 1 ("Active Cell:Active Column Number")
          # "Prepares the report string for the checked folders"
          n106 = Increment(x=w305) -> (x+1=w303:i32)
          n107 = Increment(x=w303) -> (x+1=w304:i32)
          n108 = property on="Tree" class="Tree (strict)"(error in=w315, "Active Item Tag"=w309, "ActiveColNum"=w305, "ActiveColNum"=w303, "ActiveColNum"=w304) -> (error out=w314:errorcluster, "Active Item Tag"=w308:string, "Cell String"=w312:string, "Cell String"=w311:string, "Cell String"=w310:string)  [unwired: 1 in, 1 out]
          n109 = Format Into String(format string="Path: %s \nLast Modified: %s\nType: %s\nSize: %s\n<------------------------------------------------------------------------>\\n", error in=w314, w308, w312, w311, w310) -> (resulting string=w307:string, error out=w313:errorcluster)  [unwired: 1 in]
        }
        n110 = Concatenate Strings(w296) -> (w299:string)
        n111 = Bundle By Name(cluster=w302, "Report String"=w299) -> (w300:T2)
      }
      frame "/***Search Operation***/" {
      }
      frame "Search Results" {
        # "Extracts the tags of the folders who match with the search string"
        n112 = Unbundle By Name(w328) -> ("Folder Items"=w327:T3[], "Search String"=w324:string)
        n113 = for {
          tunnel: w327 -> [w340] mode=indexing
          tunnel: [w338] -> w322 mode=indexing if=w339
          tunnel: w324 -> [w336]
          shift-right: [w335] -> w321
          shift-left: w325 -> [w335]
          # "Extracts the tag if folder name matches with search string"
          n114 = Unbundle By Name(w340) -> ("Child Tag"=w338:string, "Left Cell String"=w337:string)
          n115 = To Lower Case(string=w336) -> (all lower case string=w333:string)
          n116 = To Lower Case(string=w337) -> (all lower case string=w334:string)
          n117 = Equal?(x=w334, y=w333) -> (x = y?=w339:bool)
        }
        n118 = Empty Array?(array=w322) -> (empty?=w319:bool)
        n119 = case shown="True" w319 {
          tunnel: [w329 w332] -> w320
          tunnel: w321 -> [w329 w332]
          frame False {
          }
          frame True {
            # "Searched folder does not exist"
            n120 = One Button Dialog(message="Folder does not exist", button name ("OK")="OK") -> ()  [unwired: 1 out]
          }
        }
        n121 = Bundle By Name(cluster=w328, "Search Results"=w322) -> (w326:T2)
      }
      frame "Expand Search" {
        # "Makes the searched folder visible and open in the tree"
        n122 = Unbundle By Name(w347) -> ("Search Results"=w346:string[])
        n123 = for {
          shift-right: [w352] -> w342
          shift-left: w345 -> [w350]
          tunnel: w346 -> [w348] mode=indexing
          # "Makes the folder visible and open"
          n124 = invoke on="Tree" class="Tree (strict)" method="Open/Close.Ensure Visible"(error in=w350, "tag"=w348) -> (error out=w349:errorcluster)  [unwired: 2 in, 3 out]
          n125 = invoke on="Tree" class="Tree (strict)" method="Open/Close.Item"(error in=w349, "tag"=w348, "Open"=TRUE ("Open?")) -> (error out=w352:errorcluster)  [unwired: 2 in, 4 out]
        }
        n126 = property on="Search Bar" class="CmbBox"(error in=w342, "Text.Text"="") -> (error out=w341:errorcluster)  [unwired: 1 in, 1 out]
      }
      frame "/***Copy Opearation***/" {
      }
      frame "Selected Tags" {
        # "Reads the tags of the selected files/folders"
        n127 = Variant To Data(error in=w363, type=string[] [] ("NewVal"), Variant=w362) -> (data=w358:string[], error out=w357:errorcluster)
        n128 = Bundle By Name(cluster=w359, "Selected tags"=w358) -> (w360:T2)
      }
      frame "Trigger Copy" {
        # "Triggers the copy operation if any of the files is selected"
        n129 = Unbundle By Name(w369) -> ("Files Selected"=w368:string[])
        n130 = Empty Array?(array=w368) -> (empty?=w365:bool)
        n131 = case shown="False" w365 {
          tunnel: [w371 w376] -> w366
          tunnel: w367 -> [w372 w376]
          frame False {
            # "Files selected"
            n132 = call "Queue Driver.vi"("Array of Elements"=T1[] [{"State"="Copy Files", "Data"=variant}, {"State"="Repopulate Tree", "Data"=variant}], "Error In"=w372, "Queue Operation"=Queue_Operation."Enqueue N") -> ("Error Out"=w371:errorcluster)  [unwired: 11 in, 1 out]
          }
          frame True {
            # "No files are selected"
            n133 = One Button Dialog(message="Select files to Copy", button name ("OK")="OK") -> ()  [unwired: 1 out]
          }
        }
      }
      frame "Selected Files" {
        # "Separates the selected files"
        n134 = Unbundle By Name(w382) -> ("Selected tags"=w380:string[])
        n135 = for {
          tunnel: w380 -> [w386] mode=indexing
          shift-right: [w387] -> w381
          shift-left: w383 -> [w388]
          tunnel: [w384] -> w378 mode=indexing if=w385
          # "Checks id the selected items are files and store it"
          n136 = property on="Tree" class="Tree (strict)"(error in=w388, "Active Item Tag"=w386) -> (error out=w387:errorcluster, "Active Item Tag"=w384:string, "Child-Only?"=w385:bool)  [unwired: 1 in, 1 out]
        }
        n137 = Bundle By Name(cluster=w382, "Files Selected"=w378) -> (w379:T2)
      }
      frame "Copy Files" {
        # "Copies the files in the destination selected by the user"
        n138 = call "File Dialog"("error in"=w396) -> ("selected path"=w394:path, "exists"=w393:bool, "cancelled"=w392:bool, "error out"=w397:errorcluster)  [unwired: 11 in]
        n139 = case shown="True" w392 {
          tunnel: w397 -> [w406 w434]
          tunnel: [w405 w432] -> w395
          tunnel: w394 -> [w399 _]
          tunnel: w393 -> [_ _]
          tunnel: [w400 w436] -> w390
          tunnel: w391 -> [w403 w436]
          frame False {
            # "Checks if the path specified by user exists and creates the folder accordingly to perform copy operation"
            n140 = Unbundle By Name(w403) -> ("Files Selected"=w404:string[])
            n141 = for {
              shift-right: [w410] -> w405
              shift-left: w406 -> [w414]
              tunnel: w404 -> [w415] mode=indexing
              tunnel: w399 -> [w413]
              tunnel: [w407] -> w402 mode=indexing
              # "Copies the selected files"
              n142 = String To Path(string=w415) -> (path=w409:path)
              n143 = Copy(8:w414, 10:w413, 11:w409) -> (0:w412:errorcluster)  [unwired: 2 in, 2 out]
              n144 = Unbundle By Name(w412) -> ("code"=w411:i32)
              n145 = Strip Path(path=w409) -> (name=w408:string)  [unwired: 1 out]
              n146 = case shown="0, Default" w411 {
                tunnel: w412 -> [w418 w430]
                tunnel: [w417 w429] -> w410
                tunnel: w408 -> [w416 w426]
                tunnel: [TRUE FALSE] -> w407
                frame 0, Default {
                  n147 = Format Into String(format string=" %s copied successfully" ("message"), error in=w418, w416) -> (resulting string=w419:string, error out=w417:errorcluster)  [unwired: 1 in]
                  n148 = One Button Dialog(message=w419, button name ("OK")="OK") -> ()  [unwired: 1 out]
                }
                frame 10 {
                  # "File already exists in the folder"
                  n149 = call <vilib>:"Clear Errors.vi"("error in (no error)"=w430) -> ("error out"=w424:errorcluster)  [unwired: 5 in, 1 out]
                  n150 = Format Into String(format string=" %s already exists in the folder" ("message"), error in=w424, w426) -> (resulting string=w425:string, error out=w429:errorcluster)  [unwired: 1 in]
                  n151 = One Button Dialog(message=w425, button name ("OK")="OK") -> ()  [unwired: 1 out]
                }
              }
            }
            n152 = Boolean Array To Number(Boolean array=w402) -> (number=w401:u32)
            n153 = Greater Than 0?(x=w401) -> (x > 0?=w398:bool)
            n154 = Bundle By Name(cluster=w403, "Repopulate?"=w398, "New Folder Path"=w399) -> (w400:T2)
          }
          frame True {
            # "User cancelled the File dialog, notifies and clear the error"
            n155 = call <vilib>:"Clear Errors.vi"("error in (no error)"=w434, "specific error code to clear (0: all)"=43) -> ("error out"=w432:errorcluster)  [unwired: 4 in, 1 out]
            n156 = One Button Dialog(message="Copy operation cancelled by user.", button name ("OK")="Ok") -> ()  [unwired: 1 out]
          }
        }
      }
      frame "Repopulate Tree" {
        # "If destination path is inside the root path the tree repopulates to display the newly added folder in the tree"
        n157 = Unbundle By Name(w449) -> ("Repopulate?"=w438:bool, "New Folder Path"=w442:path, "Path In"=w448:path)
        n158 = Path To String(path=w442) -> (string=w443:string)
        n159 = Path To String(path=w448) -> (string=w446:string)
        n160 = Search and Replace String(input string=w443, search string=w446, error in=w447) -> (number of replacements=w444:i32, error out=w445:errorcluster)  [unwired: 5 in, 2 out]
        n161 = Greater Than 0?(x=w444) -> (x > 0?=w439:bool)
        n162 = And(x=w438, y=w439) -> (x .and. y?=w437:bool)
        n163 = case shown="True" w437 {
          tunnel: w445 -> [w450 w453]
          tunnel: [w450 w452] -> w440
          frame False {
          }
          frame True {
            # "Repopulates the tree"
            n164 = call "Queue Driver.vi"("Array of Elements"=T1[] [{"State"="Save Node Status", "Data"=variant}, {"State"="Clear Tree", "Data"=variant}, {"State"="Recursive List", "Data"=variant}, {"State"="Folder Items", "Data"=variant}, {"State"="File Items", "Data"=variant}, {"State"="Add Folder Items", "Data"=variant}, {"State"="Open Nodes", "Data"=variant}, {"State"="Add File Items", "Data"=variant}], "Error In"=w453, "Queue Operation"=Queue_Operation."Enqueue N") -> ("Error Out"=w452:errorcluster)  [unwired: 11 in, 1 out]
          }
        }
      }
      frame "/***Sort Operation***/" {
      }
      frame "Sort Type" {
        # "Decides the type of sort to be performed"
        n165 = Variant To Data(error in=w469, type=0 ("Case Sensitivity"), Variant=w467) -> (data=w466:i32, error out=w460:errorcluster)
        n166 = Unbundle By Name(w464) -> ("Time Flag"=w463:i16, "Type Flag"=w462:i16, "Size Flag"=w461:i16)
        n167 = case shown="2" w466 {
          selector: w466 -> [_ w475 w484 w492]
          tunnel: [w471 w478 w486 w494] -> w465
          tunnel: w464 -> [w471 w479 w487 w495]
          tunnel: w463 -> [_ _ w480 _]
          tunnel: w462 -> [_ _ _ w488]
          tunnel: w461 -> [_ w476 _ _]
          tunnel: w460 -> [w470 w477 w485 w493]
          tunnel: [w470 w477 w485 w493] -> w459
          frame Default {
          }
          frame 3 {
            # "Size sort"
            n168 = Not Equal To 0?(x=w476) -> (x != 0?=w472:bool)
            n169 = Not(x=w472) -> (.not. x?=w473:bool)
            n170 = Boolean To (0,1)(Boolean=w473) -> (0, 1=w474:i16)
            n171 = Bundle By Name(cluster=w479, "Reverse?"=w472, "Size Flag"=w474, "Sort Header"=w475) -> (w478:T2)
          }
          frame 1 {
            # "Last modified Sort"
            n172 = Not Equal To 0?(x=w480) -> (x != 0?=w483:bool)
            n173 = Not(x=w483) -> (.not. x?=w481:bool)
            n174 = Boolean To (0,1)(Boolean=w481) -> (0, 1=w482:i16)
            n175 = Bundle By Name(cluster=w487, "Reverse?"=w483, "Time Flag"=w482, "Sort Header"=w484) -> (w486:T2)
          }
          frame 2 {
            # "File type sort"
            n176 = Not Equal To 0?(x=w488) -> (x != 0?=w491:bool)
            n177 = Not(x=w491) -> (.not. x?=w489:bool)
            n178 = Boolean To (0,1)(Boolean=w489) -> (0, 1=w490:i16)
            n179 = Bundle By Name(cluster=w495, "Reverse?"=w491, "Type Flag"=w490, "Sort Header"=w492) -> (w494:T2)
          }
        }
      }
      frame "Sort" {
        # "Sort the contents of the tree"
        n180 = Unbundle By Name(w499) -> ("Sort Header"=w498:i32, "Reverse?"=w497:bool)
        n181 = invoke on="Tree" class="Tree (strict)" method="Edit Tree Items.Sort Children"(error in=w503, "tag"="" ("Tag"), "Sort Column"=w498, "Sort Recursively"=TRUE ("Sort Recursively?"), "Reverse Order"=w497) -> (error out=w502:errorcluster)  [unwired: 3 in, 7 out]
      }
      frame "/***Open/Close Nodes***/" {
      }
      frame "Save Node Status" {
        # "Saves the node status which will be used to repopulate the tree"
        n182 = Unbundle By Name(w512) -> ("All Folders"=w507:path[])
        n183 = Path To String(path=w507) -> (string=w511:string[])
        n184 = for {
          shift-right: [w517] -> w513
          shift-left: w514 -> [w518]
          tunnel: w511 -> [w516] mode=indexing
          tunnel: [w515] -> w509 mode=indexing
          n185 = property on="Tree" class="Tree (strict)"(error in=w518, "Active Item Tag"=w516) -> (error out=w517:errorcluster, "Open?"=w515:bool)  [unwired: 1 in, 1 out]
        }
        n186 = Bundle By Name(cluster=w512, "Nodes"=w507, "Open? State"=w509) -> (w510:T2)
      }
      frame "Open Nodes" {
        # "Open or close the node based on the saved status"
        n187 = Unbundle By Name(w524) -> ("Nodes"=w523:path[], "Open? State"=w521:bool[])
        n188 = Path To String(path=w523) -> (string=w519:string[])
        n189 = for {
          shift-right: [w529] -> w525
          shift-left: w522 -> [w528]
          tunnel: w519 -> [w527] mode=indexing
          tunnel: w521 -> [w526] mode=indexing
          # "Opens/ Closes the nodes"
          n190 = invoke on="Tree" class="Tree (strict)" method="Open/Close.Item"(error in=w528, "tag"=w527, "Open"=w526) -> (error out=w529:errorcluster)  [unwired: 2 in, 4 out]
        }
      }
      frame "Expand or Collapse" {
        # "Opens or closes all the folder"
        n191 = Unbundle By Name(w532) -> ("Expand?"=w531:bool)
        n192 = invoke on="Tree" class="Tree (strict)" method="Open/Close.Open/Close All"(error in=w534, "Open"=w531) -> (error out=w533:errorcluster)  [unwired: 2 in, 3 out]
      }
      frame "/***Error***/" {
      }
      frame "Error" {
        # "Handles the consumer error based on user response"
        n193 = Unbundle By Name(w544) -> ("code"=w546:i32, "source"=w545:string)
        n194 = call <vilib>:"Clear Errors.vi"("error in (no error)"=w544) -> ("error out"=w551:errorcluster)  [unwired: 5 in, 1 out]
        n195 = Format Into String(format string="Error occurred in state \"%s\"!!\nError Code: %d\nError Source: %s\n\nDo you wish to continue?", error in=w551, w543, w546, w545) -> (resulting string=w549:string, error out=w541:errorcluster)  [unwired: 1 in]
        n196 = Two Button Dialog(message=w549, 1:"Exit" ("F button name (\"Cancel\")"), 2:"Continue" ("T button name (\"OK\")")) -> (T button?=w542:bool)
        n197 = case shown="False" w542 {
          tunnel: w541 -> [w554 w556]
          tunnel: [w555 w556] -> w540
          frame False {
            # "Triggers to stop the VI"
            n198 = call "Queue Driver.vi"("Array of Elements"=T1[] [{"State"="Exit", "Data"=variant}], "Error In"=w554, "Queue Operation"=Queue_Operation."Enstack N") -> ("Error Out"=w555:errorcluster)  [unwired: 11 in, 1 out]
          }
          frame True {
          }
        }
      }
      frame "Producer Error" {
        # "Handles the producer error based on user response"
        n199 = Variant To Data(error in=w568, type=T6 {"status"=FALSE, "code"=0, "source"=""} ("error out"), Variant=w559) -> (data=w557:T6, error out=w560:errorcluster)
        n200 = Unbundle By Name(w557) -> ("code"=w562:i32, "source"=w561:string)
        n201 = Format Into String(format string="Error occurred in producer loop\nError Code: %d\nError Source: %s\n\nDo you wish to continue?", error in=w560, w562, w561) -> (resulting string=w571:string, error out=w566:errorcluster)  [unwired: 1 in]
        n202 = Two Button Dialog(message=w571, 1:"Exit" ("F button name (\"Cancel\")"), 2:"Continue" ("T button name (\"OK\")")) -> (T button?=w567:bool)
        n203 = case shown="False" w567 {
          tunnel: w566 -> [w575 w577]
          tunnel: [w576 w577] -> w565
          frame False {
            # "Triggers to stop the VI"
            n204 = call "Queue Driver.vi"("Array of Elements"=T1[] [{"State"="Exit", "Data"=variant}], "Error In"=w575, "Queue Operation"=Queue_Operation."Enstack N") -> ("Error Out"=w576:errorcluster)  [unwired: 11 in, 1 out]
          }
          frame True {
          }
        }
      }
      frame "/***Exit***/" {
      }
      frame "Exit" {
        # "Releases the queue and stops the consumer loop"
        n205 = call "Queue Driver.vi"("Error In"=w590, "Queue Operation"=Queue_Operation."Flush") -> ("Error Out"=w589:errorcluster)  [unwired: 12 in, 1 out]
        n206 = call "Queue Driver.vi"("Error In"=w589, "Queue Operation"=Queue_Operation."Release") -> ("Error Out"=w588:errorcluster)  [unwired: 12 in, 1 out]
        n207 = Unbundle By Name(w583) -> ("Stop Event"=w582:refnum<user-event>)
        n208 = Generate User Event(user event=w582, event data cluster=TRUE ("event data"), error in=w588) -> (error out=w584:errorcluster)  [unwired: 1 in, 1 out]
      }
      frame Default {
        n209 = Wait (ms)(milliseconds to wait=u32 10) -> ()  [unwired: 1 out]
      }
    }
  }
  n210 = while {
    shift-right: [w595] -> w19
    shift-left: w20 -> [w599]
    tunnel: w10 -> [w597]
    tunnel: [w596] -> w7
    stop <- w598 stop-if-true
    # "Producer Loop"
    n211 = case shown="No Error" w599 {
      selector: w599 -> [w605 w684]
      tunnel: [w603 FALSE ("Stop")] -> w598
      tunnel: w597 -> [w602 w677]
      tunnel: [w601 w681] -> w595
      tunnel: [w600 w677] -> w596
      frame No Error {
        # "Performs the file explorer operations"
        n212 = event shown="[0] Timeout" {
          selector: w602 -> [_ _ _ _ _ _ _ _ _ _]
          dyn-events: [_ _ _ _ _ _ _ _ _ _] -> w600
          timeout: 100 -> [_ _ _ _ _ _ _ _ _ _]
          tunnel: w605 -> [w607 w616 w618 w630 w643 w651 w657 w662 w672 w676]
          tunnel: [w607 w615 w619 w629 w642 w650 w657 w661 w671 w676] -> w601
          tunnel: [FALSE ("Stop") FALSE ("Discard?") FALSE ("Discard?") FALSE ("Discard?") FALSE ("Discard?") FALSE ("Discard?") w655 FALSE ("Discard?") w669 w675] -> w603
          event Timeout {
            # "Waits for any of the events to occur"
            n213 = event-data() -> ()  [unwired: 1 in, 1 out]
          }
          event "Top Level folder path": Value Change {
            # "Sends the path specified by the user"
            n214 = event-data() -> ("NewVal"=w613:path)  [unwired: 1 in]
            n215 = To Variant(anything=w613) -> (Variant=w612:variant)
            n216 = Bundle By Name(cluster=T1 {"State"="", "Data"=variant} ("Enqueue Element"), "Data"=w612, "State"="Read Path") -> (w610:T1)
            n217 = Build Array(w610) -> (w609:T1[])
            n218 = call "Queue Driver.vi"("Array of Elements"=w609, "Error In"=w616, "Queue Operation"=Queue_Operation."Enqueue N") -> ("Error Out"=w615:errorcluster)  [unwired: 11 in, 1 out]
          }
          event "Tree": Value Change {
            # "Sends the tags of the selected files"
            n219 = event-data() -> ("NewVal"=w627:string[])  [unwired: 1 in]
            n220 = To Variant(anything=w627) -> (Variant=w624:variant)
            n221 = Bundle By Name(cluster=T1 {"State"="", "Data"=variant} ("Enqueue Element"), "Data"=w624, "State"="Selected Tags") -> (w625:T1)
            n222 = Build Array(w625, T1 {"State"="Selected Files", "Data"=variant} ("element")) -> (w626:T1[])
            n223 = call "Queue Driver.vi"("Array of Elements"=w626, "Error In"=w618, "Queue Operation"=Queue_Operation."Enqueue N") -> ("Error Out"=w619:errorcluster)  [unwired: 11 in, 1 out]
          }
          event "Tree": Mouse Down {
            # "Sends the mouse down co-ordinates"
            n224 = event-data() -> ("Coords"=w638:T5)  [unwired: 1 in]
            n225 = To Variant(anything=w638) -> (Variant=w634:variant)
            n226 = Bundle By Name(cluster=T1 {"State"="", "Data"=variant} ("Enqueue Element"), "Data"=w634, "State"="Tree Mouse Down") -> (w635:T1)
            n227 = Build Array(w635) -> (w636:T1[])
            n228 = call "Queue Driver.vi"("Array of Elements"=w636, "Error In"=w630, "Queue Operation"=Queue_Operation."Enqueue N") -> ("Error Out"=w629:errorcluster)  [unwired: 11 in, 1 out]
          }
          event "Search Bar": Value Change {
            # "Sends the searched string and performs the expand operation"
            n229 = event-data() -> ("NewVal"=w644:string)  [unwired: 1 in]
            n230 = To Variant(anything=w644) -> (Variant=w649:variant)
            n231 = Bundle By Name(cluster=T1 {"State"="", "Data"=variant} ("Enqueue Element"), "Data"=w649, "State"="Read Search String") -> (w648:T1)
            n232 = Build Array (concatenate)(w648, T1[] [{"State"="Search Results", "Data"=variant}, {"State"="Expand Search", "Data"=variant}] ("appended array")) -> (w647:T1[])
            n233 = call "Queue Driver.vi"("Array of Elements"=w647, "Error In"=w643, "Queue Operation"=Queue_Operation."Enqueue N") -> ("Error Out"=w642:errorcluster)  [unwired: 11 in, 1 out]
          }
          event "Copy": Value Change {
            # "Triggers the copy operation"
            n234 = event-data() -> ()  [unwired: 1 in, 1 out]
            n235 = call "Queue Driver.vi"("Array of Elements"=T1[] [{"State"="Trigger Copy", "Data"=variant}], "Error In"=w651, "Queue Operation"=Queue_Operation."Enqueue N") -> ("Error Out"=w650:errorcluster)  [unwired: 11 in, 1 out]
          }
          event "Top Level folder path": Key Down? {
            w656 = TRUE ("Discard?")
            n236 = event-data() -> ()  [unwired: 1 in, 1 out]
            n237 = Not(x=w656) -> (.not. x?=w655:bool)
            n238 = event-data("Discard?"=w656) -> ()  [unwired: 1 in, 1 out]
          }
          event "Expand/Collapse All": Value Change {
            # "Sends the status of the Expand/Collapse boolean"
            n239 = event-data() -> ("NewVal"=w663:bool)  [unwired: 1 in]
            n240 = To Variant(anything=w663) -> (Variant=w666:variant)
            n241 = Bundle By Name(cluster=T1 {"State"="", "Data"=variant} ("Enqueue Element"), "Data"=w666, "State"="Read Expand") -> (w667:T1)
            n242 = Build Array (concatenate)(w667, T1[] [{"State"="Expand or Collapse", "Data"=variant}] ("appended array")) -> (w668:T1[])
            n243 = call "Queue Driver.vi"("Array of Elements"=w668, "Error In"=w662, "Queue Operation"=Queue_Operation."Enqueue N") -> ("Error Out"=w661:errorcluster)  [unwired: 11 in, 1 out]
          }
          event Panel Close? {
            w674 = TRUE ("Discard?")
            # "Triggers the consumer loop to stop"
            n244 = event-data() -> ()  [unwired: 1 in, 1 out]
            n245 = call "Queue Driver.vi"("Array of Elements"=T1[] [{"State"="Exit", "Data"=variant}], "Error In"=w672, "Queue Operation"=Queue_Operation."Enstack N") -> ("Error Out"=w671:errorcluster)  [unwired: 11 in, 1 out]
            n246 = Not(x=w674) -> (.not. x?=w669:bool)
            n247 = event-data("Discard?"=w674) -> ()  [unwired: 1 in, 1 out]
          }
          event User Event {
            # "Stops the producer loop"
            n248 = event-data() -> ("Stop"=w675:bool)  [unwired: 1 in]
          }
        }
      }
      frame Error {
        # "Sends the error to the consumer loop to handle"
        n249 = To Variant(anything=w684) -> (Variant=w686:variant)
        n250 = Bundle By Name(cluster=T1 {"State"="", "Data"=variant} ("Enqueue Element"), "State"="Producer Error", "Data"=w686) -> (w682:T1)
        n251 = call <vilib>:"Clear Errors.vi"("error in (no error)"=w684) -> ("error out"=w683:errorcluster)  [unwired: 5 in, 1 out]
        n252 = Build Array(w682) -> (w679:T1[])
        n253 = call "Queue Driver.vi"("Array of Elements"=w679, "Error In"=w683, "Queue Operation"=Queue_Operation."Enqueue N") -> ("Error Out"=w681:errorcluster)  [unwired: 11 in, 1 out]
      }
    }
  }
  n254 = Unregister For Events(event registration refnum=w7, error in=w19) -> (error out=w9:errorcluster)
  n255 = Destroy User Event(user event=w4, error in=w9) -> (error out=w8:errorcluster)
  n256 = Merge Errors(w8, w13) -> (→"Error Out":errorcluster)
